vi "Calibration Factors (SubVI).vi"(1 "IP List":string[][](array[string])) -> (0 "Calibration Factors":dbl[](array[numeric]))   [LabVIEW 2018]
panel:
  in  "Empty Array":dbl[](array[numeric])
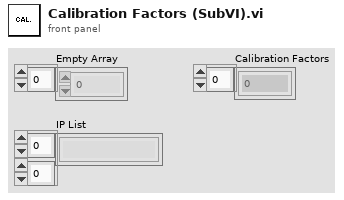
[diagram p1: front panel]
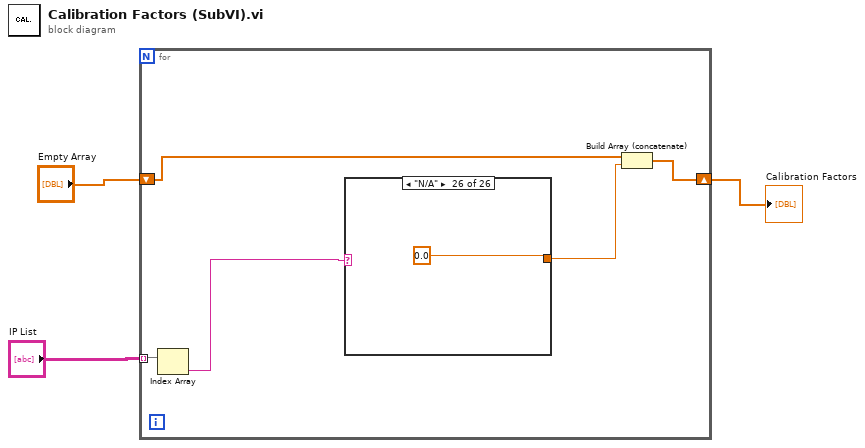
[diagram p0: block diagram]
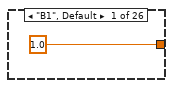
[diagram p2: hidden frame]
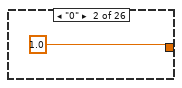
[diagram p3: hidden frame]
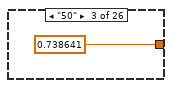
[diagram p4: hidden frame]
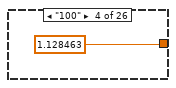
[diagram p5: hidden frame]
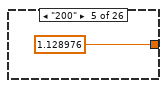
[diagram p6: hidden frame]
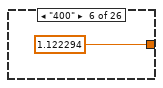
[diagram p7: hidden frame]
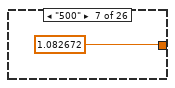
[diagram p8: hidden frame]
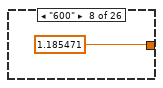
[diagram p9: hidden frame]
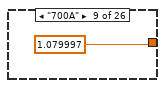
[diagram p10: hidden frame]
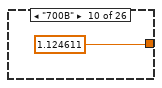
[diagram p11: hidden frame]
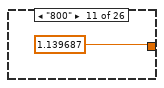
[diagram p12: hidden frame]
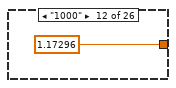
[diagram p13: hidden frame]
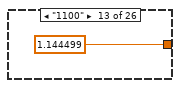
[diagram p14: hidden frame]
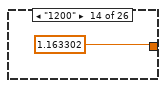
[diagram p15: hidden frame]
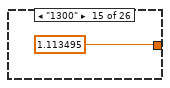
[diagram p16: hidden frame]
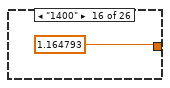
[diagram p17: hidden frame]
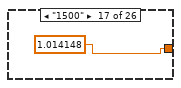
[diagram p18: hidden frame]
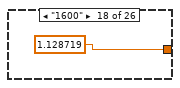
[diagram p19: hidden frame]
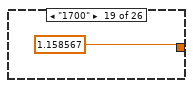
[diagram p20: hidden frame]
diagram:
  n1 = for {
    tunnel: "IP List" -> [w8] mode=indexing
    shift-right: [w7] -> w3
    shift-left: "Empty Array" -> [w6]
    n2 = Index Array(array=w8) -> (element=w5:string)  [unwired: 1 in]
    n3 = case shown="\"N/A\"" w5 {
      tunnel: [1.0 1.0 0.738641 1.128463 1.128976 1.122294 1.082672 1.185471 1.079997 1.124611 1.139687 1.17296 1.144499 1.163302 1.113495 1.164793 1.014148 1.128719 1.158567 1.147 1.096215 1.113235 1.153563 1.082672 1.183518 0.0] -> w4
      frame "B1", Default {
      }
      frame "0" {
      }
      frame "50" {
      }
      frame "100" {
      }
      frame "200" {
      }
      frame "400" {
      }
      frame "500" {
      }
      frame "600" {
      }
      frame "700A" {
      }
      frame "700B" {
      }
      frame "800" {
      }
      frame "1000" {
      }
      frame "1100" {
      }
      frame "1200" {
      }
      frame "1300" {
      }
      frame "1400" {
      }
      frame "1500" {
      }
      frame "1600" {
      }
      frame "1700" {
      }
      frame "1800" {
      }
      frame "1900" {
      }
      frame "2000" {
      }
      frame "2100" {
      }
      frame "2300" {
      }
      frame "2400" {
      }
      frame "N/A" {
      }
    }
    n4 = Build Array (concatenate)(w6, w4) -> (w7:dbl[])
  }
  "Calibration Factors" <- w3
